vi "Test.vi"() -> ()   [LabVIEW 2013]
uses:
  Controls/saveDataOption.ctl
  Globals/measurementGlobal.vi
panel:
  in  "Input No of Blocks":i32
  in  "Input No of samples":i32
  in  "Input Sampling rate (Hz)":dbl
  in  "Save Data Option":T1
  in  "Tap Control":enum32{"Plots", "File"}(tab)
  out "Comments":string
  in  "Raw Data File Path":path
  in  "Data Acquision":T2(ring)
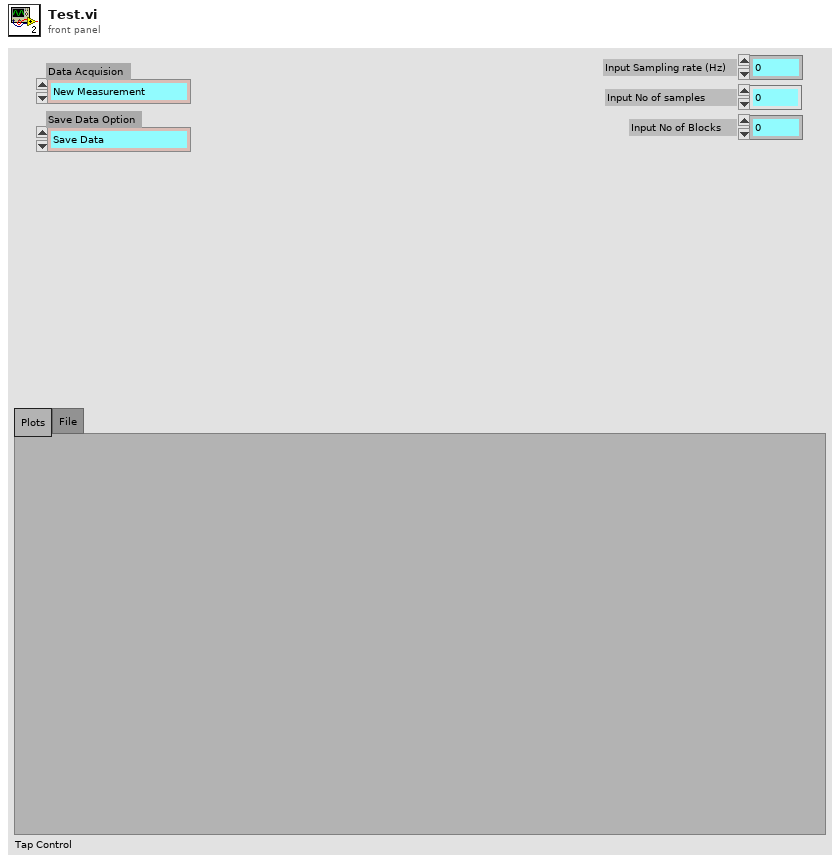
[diagram p1: front panel]
types:
  T1 = typedef "saveDataOption.ctl" = enum16{"Save Data", "Do Not Save Data"}
  T2 = enum16{"New Measurement", "Post-process Raw Data"}
  T3 = enum16{"Do Signal Processing", "No Signal Processing"}
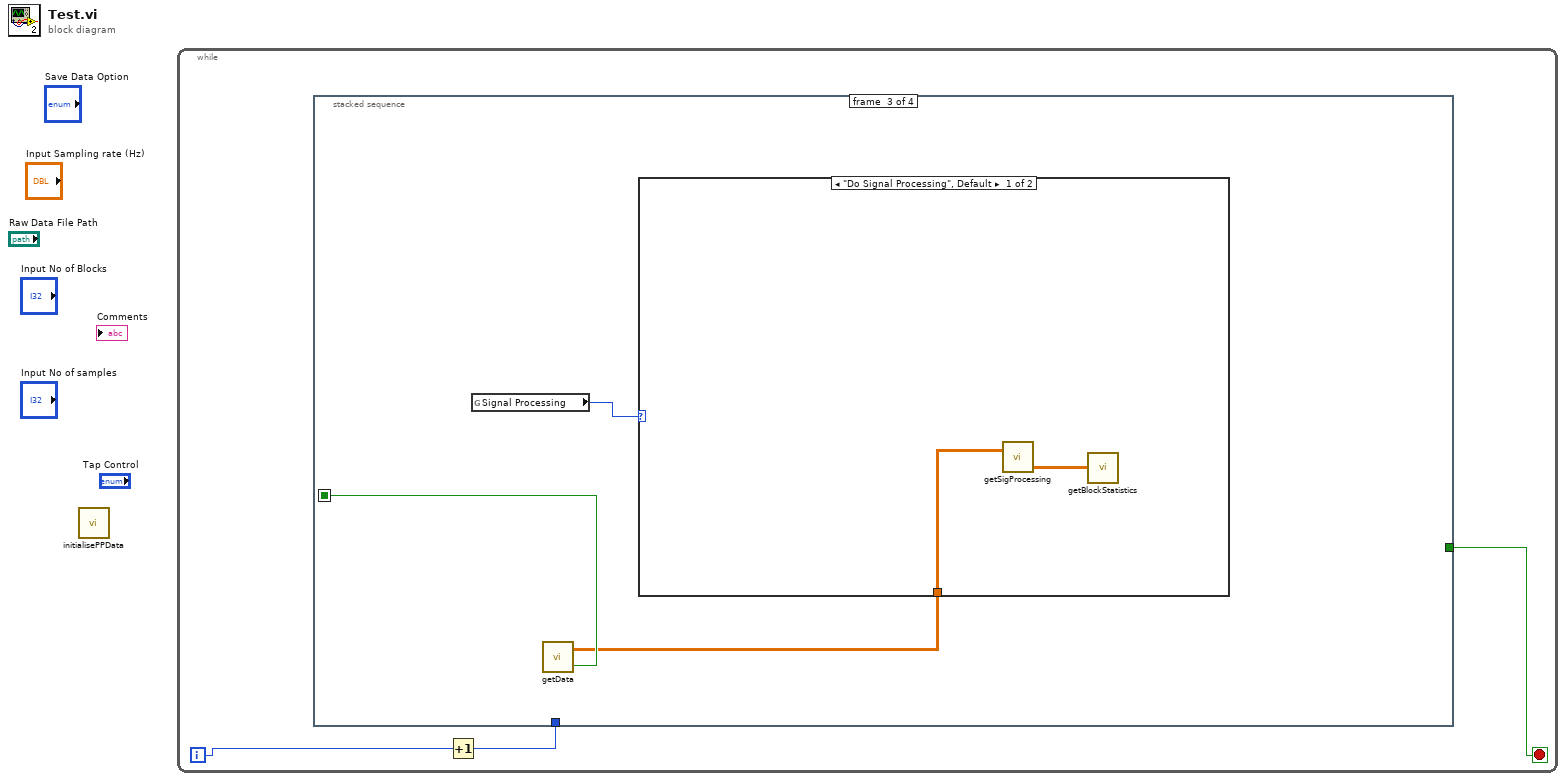
[diagram p0: block diagram]
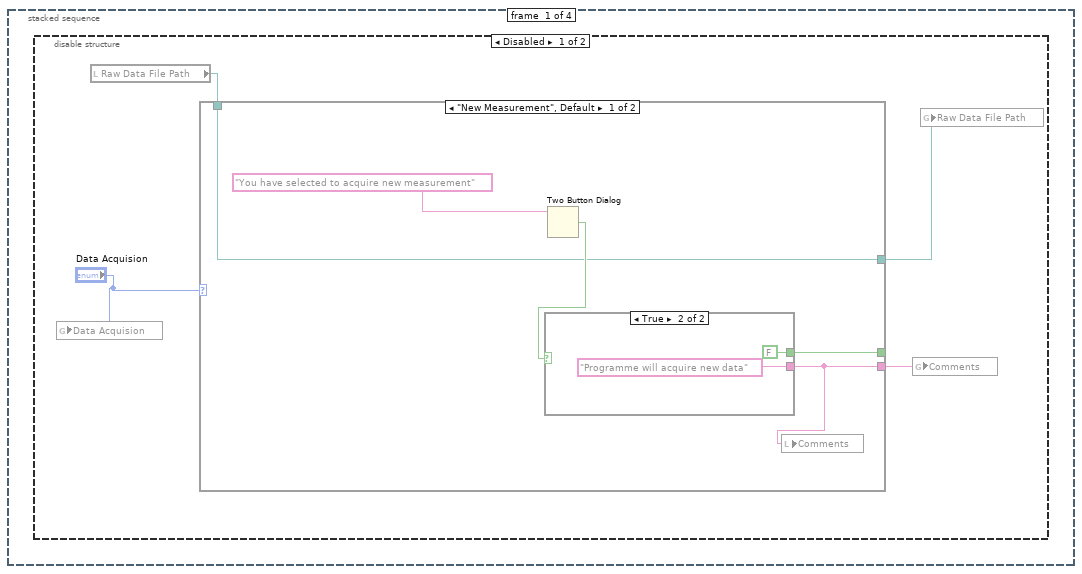
[diagram p2: hidden frame]
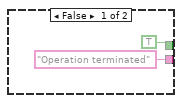
[diagram p3: hidden frame]
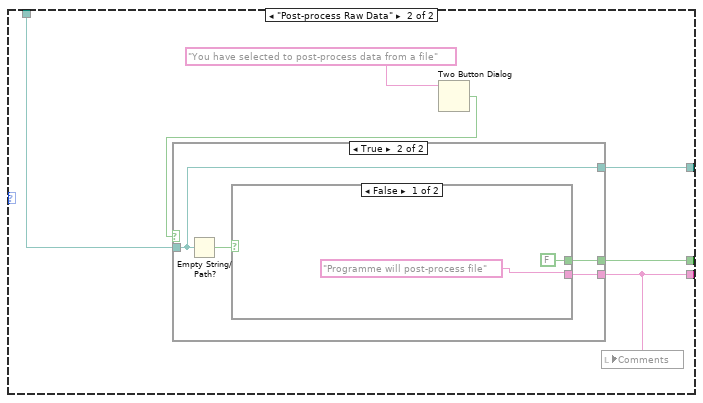
[diagram p4: hidden frame]
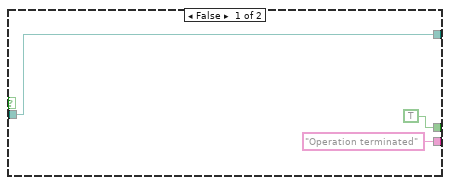
[diagram p5: hidden frame]
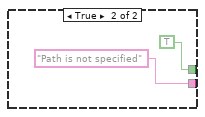
[diagram p6: hidden frame]
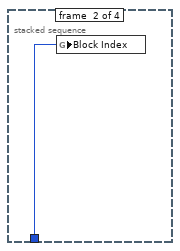
[diagram p8: hidden frame]
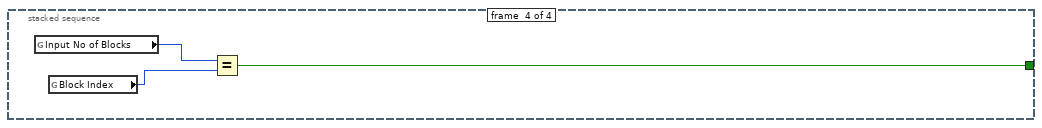
[diagram p10: hidden frame]
diagram:
  n1 = call "initialisePPData.vi"() -> ()  [unwired: 12 in]
  n2 = while {
    i -> [w3]
    stop <- w1 stop-if-true
    n3 = Increment(x=w3) -> (x+1=w2:i32)
    n4 = stacked-sequence {
      seq-local: [_ _ w37 _] -> [_ _ _ _]
      tunnel: w2 -> [_ w34 _ _]
      tunnel: [_ _ _ w40] -> w1
      frame #0 {
        n5 = disable-structure shown="Disabled" {
          frame Disabled {
            n6 = global write "measurementGlobal.vi" "Data Acquision"("Data Acquision") -> ()
            n7 = local read "Raw Data File Path"() -> (w5:path)
            n8 = case shown="\"New Measurement\", Default" "Data Acquision" {
              tunnel: [w10 w17] -> w6
              tunnel: [w9 w18] -> _
              tunnel: w5 -> [w8 w20]
              tunnel: [w8 w19] -> w4
              frame "New Measurement", Default {
                n9 = Two Button Dialog(message="You have selected to acquire new measurement") -> (T button?=w11:bool)  [unwired: 2 in]
                n10 = case shown="True" w11 {
                  tunnel: ["Operation terminated" ("Comments") "Programme will acquire new data" ("Comments")] -> w10
                  tunnel: [TRUE FALSE] -> w9
                  frame False {
                  }
                  frame True {
                  }
                }
                n11 = local write "Comments"(w10) -> ()
              }
              frame "Post-process Raw Data" {
                n12 = Two Button Dialog(message="You have selected to post-process data from a file") -> (T button?=w21:bool)  [unwired: 2 in]
                n13 = case shown="True" w21 {
                  tunnel: w20 -> [w25 w27]
                  tunnel: ["Operation terminated" w28] -> w17
                  tunnel: [w25 w27] -> w19
                  tunnel: [TRUE w26] -> w18
                  frame False {
                  }
                  frame True {
                    n14 = Empty String/Path?(string/path=w27) -> (empty?=w29:bool)
                    n15 = case shown="False" w29 {
                      tunnel: ["Programme will post-process file" "Path is not specified"] -> w28
                      tunnel: [FALSE TRUE] -> w26
                      frame False {
                      }
                      frame True {
                      }
                    }
                  }
                }
                n16 = local write "Comments"(w17) -> ()
              }
            }
            n17 = global write "measurementGlobal.vi" "Comments"(w6) -> ()
            n18 = global write "measurementGlobal.vi" "Raw Data File Path"(w4) -> ()
          }
          frame Enabled {
          }
        }
      }
      frame #1 {
        n19 = global write "measurementGlobal.vi" "Block Index"(w34) -> ()
      }
      frame #2 {
        n20 = global read "measurementGlobal.vi" "Signal Processing"() -> (w36:T3)
        n21 = call "getData.vi"() -> ("Analogue Data (volts)"=w35:dbl[][], "Error Status"=w37:bool)  [unwired: 1 in]
        n22 = case shown="\"Do Signal Processing\", Default" w36 {
          tunnel: w35 -> [w39 _]
          frame "Do Signal Processing", Default {
            n23 = call "getSigProcessing.vi"("Analogue Data (volts)"=w39) -> ("Raw Signals"=w38:dbl[][])  [unwired: 2 out]
            n24 = call "getBlockStatistics.vi"("Analogue Data (volts)"=w38) -> ()  [unwired: 1 out]
          }
          frame "No Signal Processing" {
          }
        }
      }
      frame #3 {
        n25 = global read "measurementGlobal.vi" "Input No of Blocks"() -> (w42:i32)
        n26 = global read "measurementGlobal.vi" "Block Index"() -> (w41:i32)
        n27 = Equal?(x=w42, y=w41) -> (x = y?=w40:bool)
      }
    }
  }
